vi "Untitled 2.vi"(0 "Data IN":T3={"App State"="", "Connect "=FALSE, "phandle out"=0, "Axis"=[], "S ramp"=30.0, "Acceleration"=100000.0, "Initial Speed"=10.0, "Normal Open / Close"=enum."Close", "Deceleration"=100000.0, "Creep"=30.0, "Speed"=1000.0, "X Axis"={"Operating State"="", "Current Position"=0.0, "Current Speed"=0.0, "Axis State"=0, "Angle"=0.0}, "Y Axis"={"Operating State"="", "Current Position"=0.0, "Current Speed"=0.0, "Axis State"=0, "Angle"=0.0}, "Distance"=0.0, "Direct of movement"=enum."Forward", "Move Method"=enum."Continue", "Move Mode"=enum."Relative", "Angle"=enum."0", "Times"=0, "Start Time"=0.0, "Step Flag"=FALSE, "x  dist"=[], "y dist"=[], "x angle array"=[], "y angle array"=[], "index"=0.0, "big motion angle"=0.0, "big angle"=[], "xy dy speed table"=[], "x dy speed table"=[], "y dy speed table"=[], "x dy time"=[], "y dy time"=[], "xy dy time"=[], "dy Path  "=[]}, 1 "Axis":enum16{"X", "Y", "X+Y"}(ring), 3 "Rotate":bool, 5 "dynamic":bool, 9 "Array 2":T2(array[cluster]), 11 "error IN":errorcluster, 12 "DYNAMIC":T1(array[cluster]), 13 "DYNAMIC 2":T1(array[cluster]), 14 "Speed":dbl=1.0 format="%#_13g") -> (4 "Data OUT":T3={"App State"="", "Connect "=FALSE, "phandle out"=0, "Axis"=[], "S ramp"=30.0, "Acceleration"=100000.0, "Initial Speed"=10.0, "Normal Open / Close"=enum."Close", "Deceleration"=100000.0, "Creep"=30.0, "Speed"=1000.0, "X Axis"={"Operating State"="", "Current Position"=0.0, "Current Speed"=0.0, "Axis State"=0, "Angle"=0.0}, "Y Axis"={"Operating State"="", "Current Position"=0.0, "Current Speed"=0.0, "Axis State"=0, "Angle"=0.0}, "Distance"=0.0, "Direct of movement"=enum."Forward", "Move Method"=enum."Continue", "Move Mode"=enum."Relative", "Angle"=enum."0", "Times"=0, "Start Time"=0.0, "Step Flag"=FALSE, "x  dist"=[], "y dist"=[], "x angle array"=[], "y angle array"=[], "index"=0.0, "big motion angle"=0.0, "big angle"=[], "xy dy speed table"=[], "x dy speed table"=[], "y dy speed table"=[], "x dy time"=[], "y dy time"=[], "xy dy time"=[], "dy Path  "=[]}, 15 "error out":errorcluster)   [LabVIEW 2015]
uses:
  Typedef/Data2.ctl
  zauxdll-2014/zauxdll.lvlib
panel:
  out "y angle array":i32[][](array[numeric])
  out "x angle array":i32[][](array[numeric])
  # "m"
  # "m"
  # "m"
  # "m"
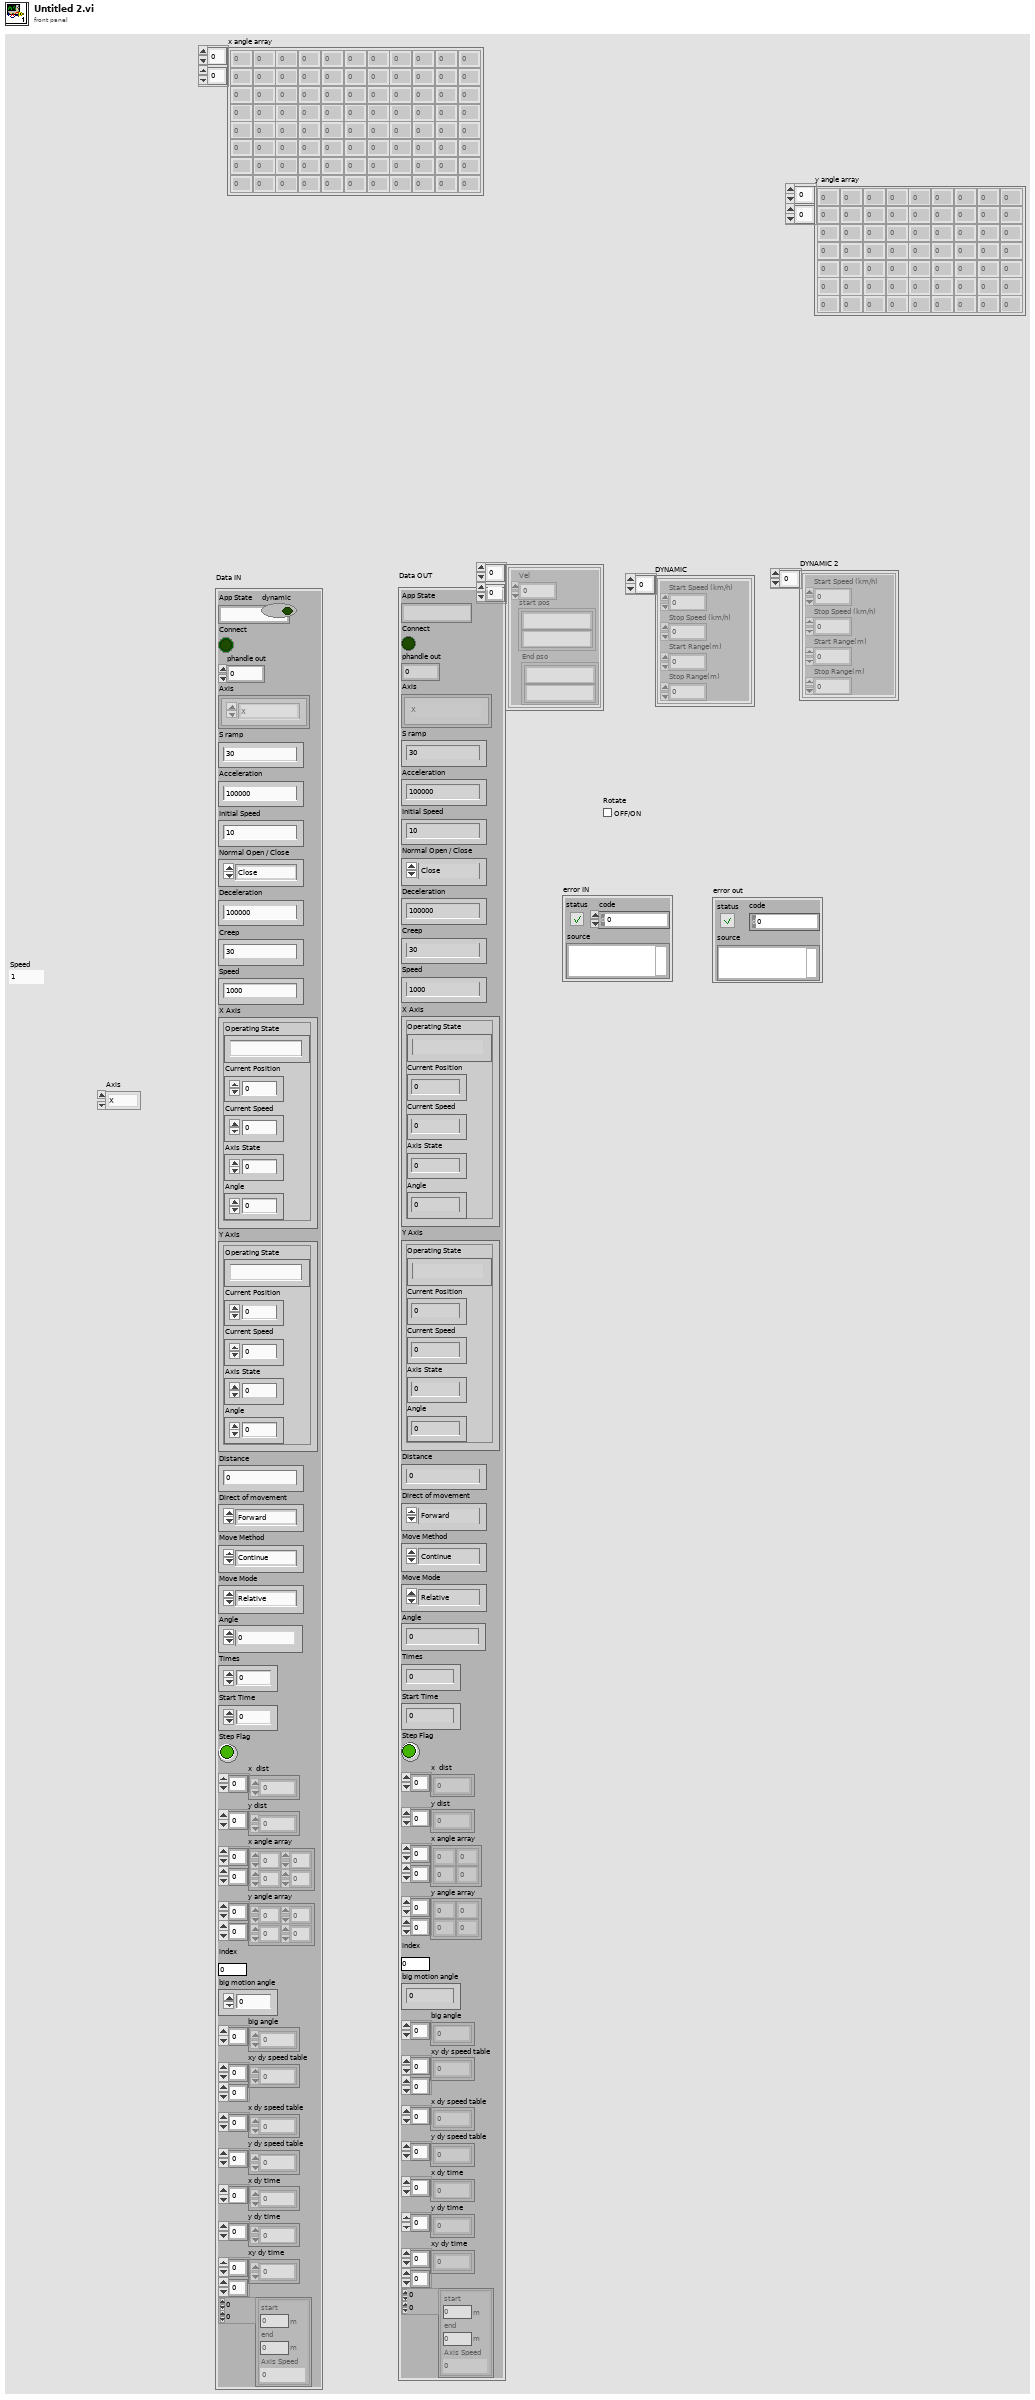
[diagram p1: front panel]
types:
  T1 = cluster{"Start Speed (km/h)":dbl, "Stop Speed (km/h) ":dbl, "Start Range(m)":dbl, "Stop Range(m)":dbl}[]
  T2 = cluster{"Vel":dbl, "start pos":cluster{string, string}, "End pso":cluster{string, string}}[][]
  T3 = typedef "Data2.ctl" = cluster{"App State":string, "Connect ":bool, "phandle out":u32, "Axis":enum16{"X", "Y", "X+Y"}[], "S ramp":dbl, "Acceleration":dbl, "Initial Speed":dbl, "Normal Open / Close":enum16{"Open", "Close"}, "Deceleration":dbl, "Creep":dbl, "Speed":dbl, "X Axis":cluster{"Operating State":string, "Current Position":dbl, "Current Speed":dbl, "Axis State":i32, "Angle":dbl}, "Y Axis":cluster{"Operating State":string, "Current Position":dbl, "Current Speed":dbl, "Axis State":i32, "Angle":dbl}, "Distance":dbl, "Direct of movement":enum16{"Forward", "Backward"}, "Move Method":enum16{"Continue", "Inching"}, "Move Mode":enum16{"Relative", "Absolute"}, "Angle":enum32{"0", "1", "10", "30", "34", "60", "90", "180", "-1", "-10"}, "Times":i32, "Start Time":dbl, "Step Flag":bool, "x  dist":dbl[], "y dist":dbl[], "x angle array":i32[][], "y angle array":i32[][], "index":dbl, "big motion angle":dbl, "big angle":dbl[], "xy dy speed table":dbl[][], "x dy speed table":dbl[], "y dy speed table":dbl[], "x dy time":dbl[], "y dy time":dbl[], "xy dy time":dbl[][], "dy Path  ":cluster{"end":dbl, "start":dbl, "Axis Speed":dbl}[][]}
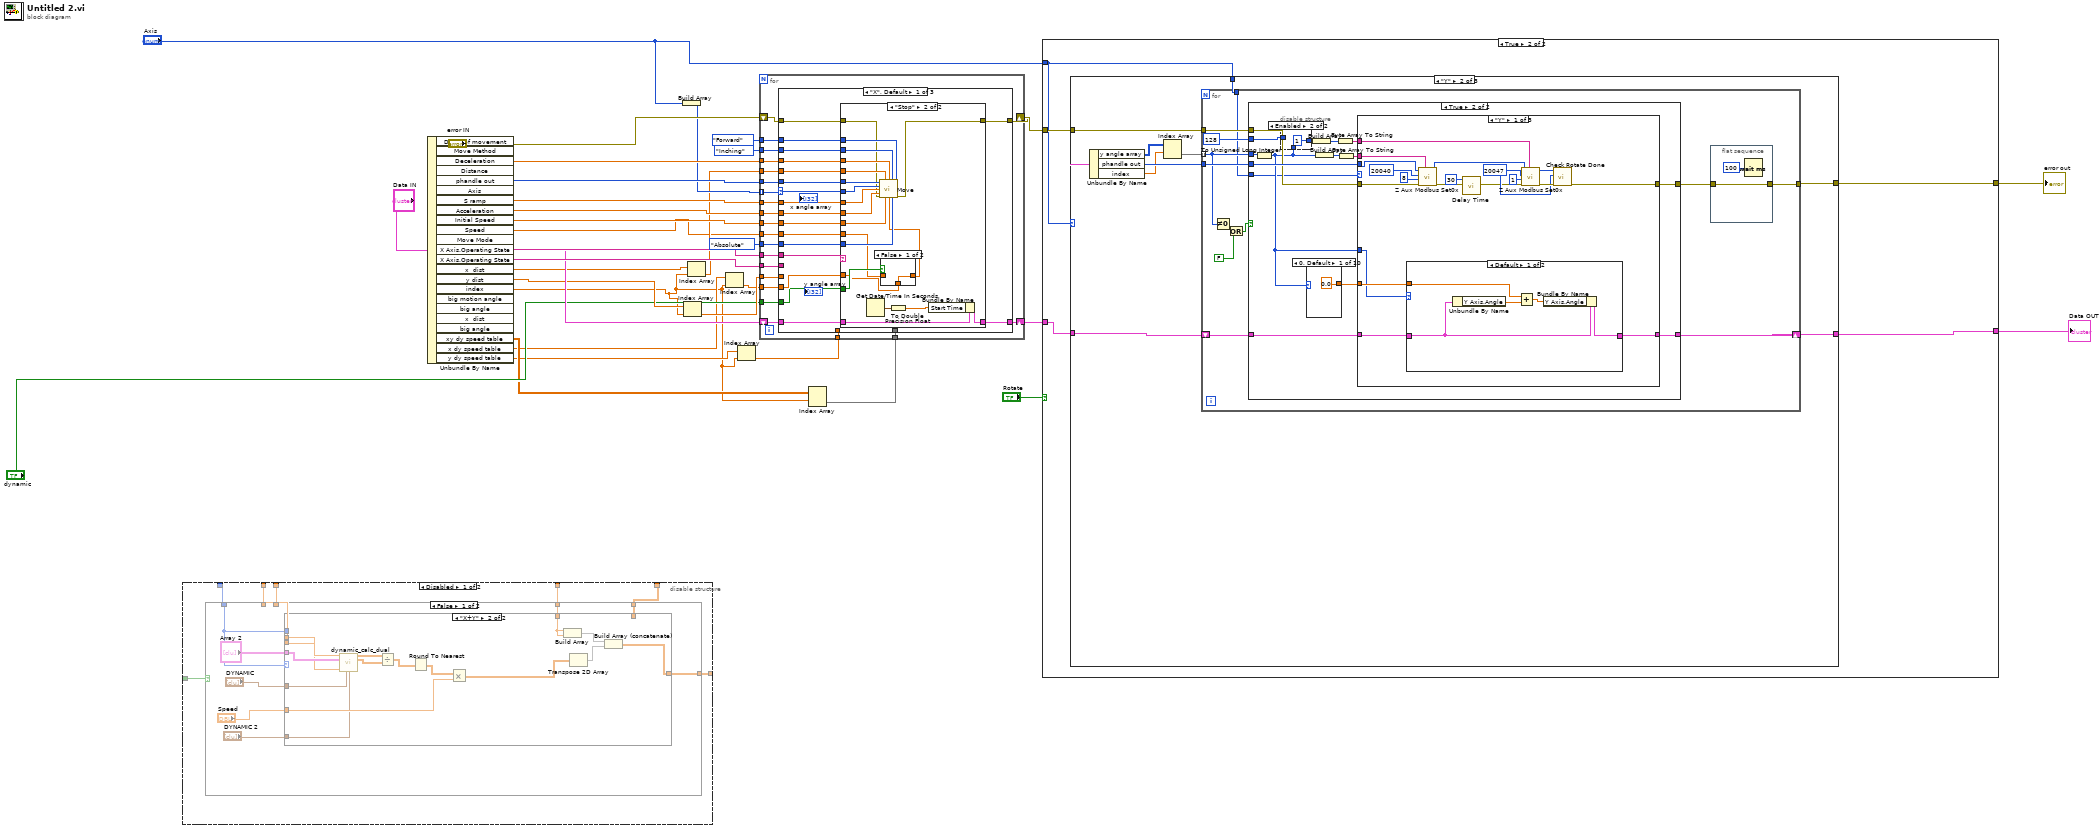
[diagram p0: block diagram]
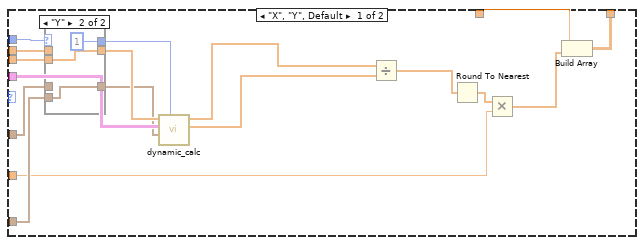
[diagram p2: hidden frame]
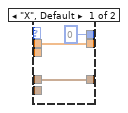
[diagram p3: hidden frame]
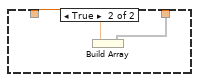
[diagram p4: hidden frame]
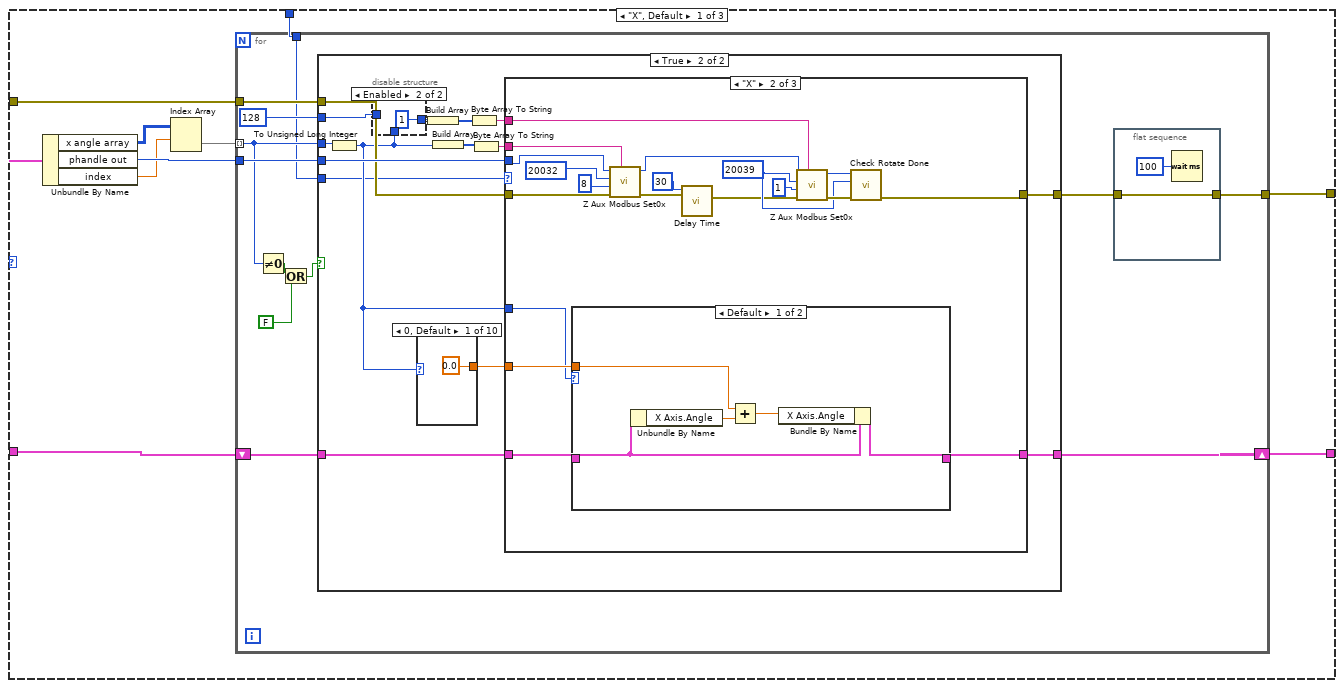
[diagram p7: hidden frame]
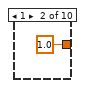
[diagram p9: hidden frame]
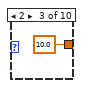
[diagram p10: hidden frame]
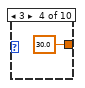
[diagram p11: hidden frame]
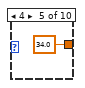
[diagram p12: hidden frame]
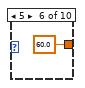
[diagram p13: hidden frame]
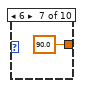
[diagram p14: hidden frame]
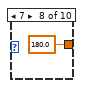
[diagram p15: hidden frame]
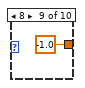
[diagram p16: hidden frame]
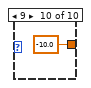
[diagram p17: hidden frame]
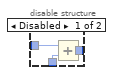
[diagram p18: hidden frame]
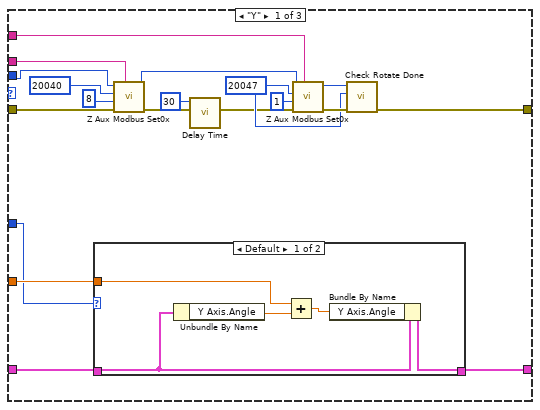
[diagram p19: hidden frame]
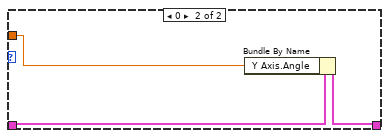
[diagram p20: hidden frame]
diagram:
  n1 = disable-structure shown="Disabled" {
    disable-tunnel: _ -> [w39 _]
    disable-tunnel: _ -> [w38 _]
    disable-tunnel: _ -> [w37 _]
    disable-tunnel: _ -> [w36 _]
    disable-tunnel: _ -> [w35 _]
    disable-tunnel: [w34 _] -> _
    disable-tunnel: [w33 _] -> _
    frame Disabled {
      n2 = case shown="False" w39 {
        tunnel: w38 -> [w43 _]
        tunnel: w37 -> [w49 w89]
        tunnel: [w48 w88] -> w34
        tunnel: w36 -> [w45 _]
        tunnel: w35 -> [w44 _]
        tunnel: [w41 _] -> w33
        frame False {
          n3 = case shown="\"X+Y\"" w43 {
            tunnel: w49 -> [w62 w78]
            tunnel: [w61 _] -> w48
            tunnel: "DYNAMIC" -> [w54 w74]
            tunnel: "Array 2" -> [w60 w87]
            tunnel: w45 -> [w58 w86]
            tunnel: w44 -> [w57 w85]
            tunnel: w43 -> [w59 _]
            tunnel: "Speed" -> [w51 w80]
            tunnel: [_ w79] -> w41
            tunnel: "DYNAMIC 2" -> [w53 w73]
            frame "X", "Y", Default {
              n4 = case shown="\"Y\"" w59 {
                tunnel: w58 -> [w69 _]
                tunnel: w57 -> [_ w72]
                tunnel: [w69 w72] -> w56
                tunnel: [0 1] -> w55
                tunnel: w54 -> [w67 _]
                tunnel: w53 -> [_ w70]
                tunnel: [w67 w70] -> w52
                frame "X", Default {
                }
                frame "Y" {
                }
              }
              n5 = call "dynamic_calc.vi"("index (row)"=w55, "DYNAMIC"=w52, "Array 2"=w60, "x  dist"=w56) -> ("time"=w64:dbl[], "Array"=w63:dbl[])  [unwired: 5 in, 1 out]
              n6 = Divide(x=w63, y=w64) -> (x/y=w50:dbl[])
              n7 = Round To Nearest(number=w50) -> (nearest integer value=w65:dbl[])
              n8 = Multiply(x=w65, y=w51) -> (x*y=w66:dbl[])
              n9 = Build Array(w62, w66) -> (w61:dbl[][])
            }
            frame "X+Y" {
              n10 = call "dynamic_calc_dual.vi"("x  dist"=w86, "Array 2"=w87, "y  dist"=w85, "DYNAMIC"=w74, "DYNAMIC 2"=w73) -> ("dist"=w84:dbl[][], "time"=w83:dbl[][])  [unwired: 9 in]
              n11 = Divide(x=w84, y=w83) -> (x/y=w82:dbl[][])
              n12 = Round To Nearest(number=w82) -> (nearest integer value=w81:dbl[][])
              n13 = Multiply(x=w81, y=w80) -> (x*y=w77:dbl[][])
              n14 = Build Array(w78, w78) -> (w75:void[])
              n15 = Transpose 2D Array(2D array=w77) -> (transposed array=w76:dbl[][])
              n16 = Build Array (concatenate)(w75, w76) -> (w79:dbl[][])
            }
          }
        }
        frame True {
          n17 = Build Array(w89) -> (w88:void[])
        }
      }
    }
    frame Enabled {
    }
  }
  n18 = Unbundle By Name("Data IN") -> ("Deceleration"=w28:dbl, "phandle out"=w32:u32, "S ramp"=w31:dbl, "Acceleration"=w30:dbl, "Initial Speed"=w29:dbl, "Speed"=w10:dbl, "X Axis.Operating State"=w27:string, "X Axis.Operating State"=w26:string, "x  dist"=w7:dbl[], "y dist"=w9:dbl[], "index"=w2:dbl, "xy dy speed table"=w5:dbl[][], "x dy speed table"=w4:dbl[], "y dy speed table"=w3:dbl[])  [unwired: 9 out]
  n19 = Build Array("Axis") -> (w16:enum16{"X", "Y", "X+Y"}[])
  n20 = Index Array(array=w9, index=w2) -> (element=w15:dbl)
  n21 = Index Array(array=w7, index=w2) -> (element=w13:dbl)
  n22 = Index Array(array=w4, index=w2) -> (element=w12:dbl)
  n23 = Index Array(array=w3, index=w2) -> (element=w1:dbl)
  n24 = Index Array(array=w5, index (row)=w2) -> (element=w8:dbl[])  [unwired: 1 in]
  n25 = for {
    tunnel: w32 -> [w111]
    tunnel: w31 -> [w110]
    tunnel: w30 -> [w109]
    tunnel: w29 -> [w108]
    tunnel: w10 -> [w107]
    tunnel: enum16{"Continue", "Inching"}."Inching" ("Move Method") -> [w106]
    tunnel: w28 -> [w105]
    tunnel: w16 -> [w104] mode=indexing
    tunnel: w13 -> [w103]
    tunnel: enum16{"Forward", "Backward"}."Forward" ("Direct of movement") -> [w102]
    tunnel: enum16{"Relative", "Absolute"}."Absolute" ("Move Mode") -> [w101]
    tunnel: w27 -> [w100]
    tunnel: w26 -> [w99]
    shift-right: [w97] -> w23
    shift-left: "Data IN" -> [w98]
    shift-right: [w95] -> w22
    shift-left: "error IN" -> [w96]
    tunnel: w15 -> [w94]
    tunnel: w12 -> [w93]
    tunnel: "dynamic" -> [w92]
    tunnel: w8 -> [w91]
    tunnel: w1 -> [w90]
    n26 = case shown="\"X\", Default" w104 {
      selector: w104 -> [w122 w165 _]
      tunnel: w111 -> [w129 w171 w219]
      tunnel: w110 -> [w128 w170 w218]
      tunnel: w109 -> [w127 w169 w217]
      tunnel: w108 -> [w126 w168 w216]
      tunnel: w107 -> [w125 w167 w215]
      tunnel: w106 -> [w124 w166 w214]
      tunnel: w105 -> [w123 w156 w213]
      tunnel: w103 -> [w120 _ w200]
      tunnel: w102 -> [w121 w164 w212]
      tunnel: w101 -> [w119 w163 w211]
      tunnel: w100 -> [w118 _ w210]
      tunnel: w99 -> [_ w162 w208]
      tunnel: w98 -> [w117 w161 w204]
      tunnel: [w116 w160 w203] -> w97
      tunnel: w96 -> [w115 w159 w202]
      tunnel: [w114 w158 w201] -> w95
      tunnel: w94 -> [_ w157 w199]
      tunnel: w93 -> [w113 _ _]
      tunnel: w92 -> [w112 w155 w197]
      tunnel: w91 -> [_ _ w196]
      tunnel: w90 -> [_ w154 _]
      frame "X", Default {
        n27 = case shown="\"Stop\"" w118 {
          tunnel: w129 -> [_ w151]
          tunnel: w128 -> [_ w150]
          tunnel: w127 -> [_ w149]
          tunnel: w126 -> [_ w148]
          tunnel: w125 -> [_ w134]
          tunnel: w124 -> [_ w147]
          tunnel: w123 -> [_ w146]
          tunnel: w122 -> [_ w145]
          tunnel: w121 -> [_ w144]
          tunnel: w120 -> [_ w143]
          tunnel: w119 -> [_ w142]
          tunnel: w117 -> [w131 w141]
          tunnel: [w131 w140] -> w116
          tunnel: w115 -> [w130 w137]
          tunnel: [w130 w136] -> w114
          tunnel: w113 -> [_ w132]
          tunnel: w112 -> [_ w135]
          frame "False", Default {
          }
          frame "Stop" {
            n28 = Get Date/Time In Seconds() -> (seconds since 1Jan1904=w139:timestamp)
            n29 = case shown="False" w135 {
              tunnel: w134 -> [_ w153]
              tunnel: [w152 w153] -> w133
              tunnel: w132 -> [w152 _]
              frame False {
              }
              frame True {
              }
            }
            n30 = call "Move.vi"("handle"=w151, "Distance"=w143, "Decel"=w146, "Move Method"=w147, "Direct of movement"=w144, "Axis"=w145, "Sramp"=w150, "Accel"=w149, "error in (no error)"=w137, "Lspeed"=w148, "Speed"=w133, "Move Mode"=w142) -> ("error out"=w136:errorcluster)  [unwired: 3 in]
            n31 = To Double Precision Float(number=w139) -> (double precision float=w138:dbl)
            n32 = Bundle By Name(cluster=w141, "Start Time"=w138) -> (w140:T3)
          }
        }
      }
      frame "Y" {
        n33 = case shown="\"Stop\"" w162 {
          tunnel: w171 -> [_ w193]
          tunnel: w170 -> [_ w192]
          tunnel: w169 -> [_ w191]
          tunnel: w168 -> [_ w190]
          tunnel: w167 -> [_ w176]
          tunnel: w166 -> [_ w189]
          tunnel: w156 -> [_ w188]
          tunnel: w165 -> [_ w187]
          tunnel: w164 -> [_ w186]
          tunnel: w157 -> [_ w185]
          tunnel: w163 -> [_ w184]
          tunnel: w161 -> [w173 w181]
          tunnel: [w173 w180] -> w160
          tunnel: w159 -> [w172 w179]
          tunnel: [w172 w178] -> w158
          tunnel: w154 -> [_ w174]
          tunnel: w155 -> [_ w177]
          frame "False", Default {
          }
          frame "Stop" {
            n34 = Get Date/Time In Seconds() -> (seconds since 1Jan1904=w183:timestamp)
            n35 = case shown="False" w177 {
              tunnel: w176 -> [_ w195]
              tunnel: [w194 w195] -> w175
              tunnel: w174 -> [w194 _]
              frame False {
              }
              frame True {
              }
            }
            n36 = To Double Precision Float(number=w183) -> (double precision float=w182:dbl)
            n37 = call "Move.vi"("handle"=w193, "Distance"=w185, "Decel"=w188, "Move Method"=w189, "Direct of movement"=w186, "Axis"=w187, "Sramp"=w192, "Accel"=w191, "error in (no error)"=w179, "Lspeed"=w190, "Speed"=w175, "Move Mode"=w184) -> ("error out"=w178:errorcluster)  [unwired: 3 in]
            n38 = Bundle By Name(cluster=w181, "Start Time"=w182) -> (w180:T3)
          }
        }
      }
      frame "X+Y" {
        w209 = "Stop" ("y")
        n39 = Build Array(w200, w199) -> (w198:dbl[])
        n40 = Equal?(x=w210, y=w209) -> (x = y?=w207:bool)
        n41 = Equal?(x=w209, y=w208) -> (x = y?=w205:bool)
        n42 = And(x=w207, y=w205) -> (x .and. y?=w206:bool)
        n43 = case shown="True" w206 {
          tunnel: w219 -> [_ w241]
          tunnel: w218 -> [_ w240]
          tunnel: w217 -> [_ w239]
          tunnel: w216 -> [_ w238]
          tunnel: w215 -> [_ w224]
          tunnel: w214 -> [_ w237]
          tunnel: w213 -> [_ w236]
          tunnel: w198 -> [_ w234]
          tunnel: w212 -> [_ w233]
          tunnel: w211 -> [_ w232]
          tunnel: w204 -> [w221 w231]
          tunnel: [w221 w230] -> w203
          tunnel: w202 -> [w220 w227]
          tunnel: [w220 w226] -> w201
          tunnel: w197 -> [_ w225]
          tunnel: w196 -> [_ w222]
          frame False {
          }
          frame True {
            n44 = case shown="False" w225 {
              tunnel: w224 -> [_ w244]
              tunnel: [w242 w243] -> w223
              tunnel: w222 -> [w242 _]
              frame False {
              }
              frame True {
                n45 = Build Array(w244, w244) -> (w243:dbl[])
              }
            }
            n46 = Get Date/Time In Seconds() -> (seconds since 1Jan1904=w229:timestamp)
            n47 = To Double Precision Float(number=w229) -> (double precision float=w228:dbl)
            n48 = for {
              tunnel: w241 -> [w257]
              tunnel: w240 -> [w256]
              tunnel: w239 -> [w255]
              tunnel: w238 -> [w254]
              tunnel: w223 -> [w253] mode=indexing
              tunnel: w237 -> [w252]
              tunnel: w236 -> [w251]
              tunnel: i32[] [0, 1] -> [w250] mode=indexing
              tunnel: w234 -> [w249] mode=indexing
              tunnel: w233 -> [w248]
              tunnel: w232 -> [w247]
              tunnel: w227 -> [w246]
              tunnel: [w245] -> w226
              n49 = call "Move.vi"("handle"=w257, "Distance"=w249, "Decel"=w251, "Move Method"=w252, "Direct of movement"=w248, "Axis"=w250, "Sramp"=w256, "Accel"=w255, "error in (no error)"=w246, "Lspeed"=w254, "Speed"=w253, "Move Mode"=w247) -> ("error out"=w245:errorcluster)  [unwired: 3 in]
            }
            n50 = Bundle By Name(cluster=w231, "Start Time"=w228) -> (w230:T3)
          }
        }
      }
    }
  }
  n51 = case shown="True" "Rotate" {
    tunnel: w23 -> [w258 w264]
    tunnel: w22 -> [w259 w263]
    tunnel: [w259 w262] -> w21
    tunnel: [w258 w261] -> w20
    tunnel: "Axis" -> [_ w260]
    frame False {
    }
    frame True {
      n52 = case shown="\"Y\"" w260 {
        tunnel: w264 -> [w271 w411 w552]
        tunnel: w263 -> [w270 w410 w556]
        tunnel: [w269 w409 w548] -> w262
        tunnel: [w268 w408 w550] -> w261
        tunnel: w260 -> [w267 w407 w555]
        frame "X", Default {
          n53 = Unbundle By Name(w271) -> ("x angle array"=w266:i32[][], "phandle out"=w273:u32, "index"=w265:dbl)
          n54 = Index Array(array=w266, index (row)=w265) -> (element=w272:i32[])  [unwired: 1 in]
          n55 = for {
            tunnel: w273 -> [w281]
            tunnel: w270 -> [w285]
            tunnel: w272 -> [w280] mode=indexing
            shift-right: [w282] -> w268
            shift-left: w271 -> [w283]
            tunnel: [w276] -> w269
            tunnel: w267 -> [w274]
            n56 = Not Equal To 0?(x=w280) -> (x != 0?=w278:bool)
            n57 = Or(x=w278, y=FALSE) -> (x .or. y?=w279:bool)
            n58 = case shown="True" w279 {
              tunnel: w281 -> [_ w304]
              tunnel: w285 -> [w289 w303]
              tunnel: u32 128 -> [_ w302]
              tunnel: w283 -> [w288 w296]
              tunnel: w280 -> [_ w295]
              tunnel: [w288 w294] -> w282
              tunnel: [w289 w293] -> w277
              tunnel: w274 -> [_ w290]
              frame False {
              }
              frame True {
                n59 = To Unsigned Long Integer(number=w295) -> (unsigned 32bit integer=w291:u32)
                n60 = disable-structure shown="Enabled" {
                  disable-tunnel: w302 -> [w317 _]
                  disable-tunnel: [w316 u32 1] -> w301
                  disable-tunnel: w291 -> [w315 _]
                  frame Disabled {
                    n61 = Add(x=w317, y=w315) -> (x+y=w316:u32)
                  }
                  frame Enabled {
                  }
                }
                n62 = case shown="0, Default" w291 {
                  tunnel: [0.0 1.0 10.0 30.0 34.0 60.0 90.0 180.0 -1.0 -10.0] -> w297
                  frame 0, Default {
                  }
                  frame 1 {
                  }
                  frame 2 {
                  }
                  frame 3 {
                  }
                  frame 4 {
                  }
                  frame 5 {
                  }
                  frame 6 {
                  }
                  frame 7 {
                  }
                  frame 8 {
                  }
                  frame 9 {
                  }
                }
                n63 = Build Array(w301) -> (w300:u32[])
                n64 = Build Array(w291) -> (w292:u32[])
                n65 = Byte Array To String(unsigned byte array=w300) -> (string=w299:string)
                n66 = Byte Array To String(unsigned byte array=w292) -> (string=w298:string)
                n67 = case shown="\"X\"" w290 {
                  tunnel: w304 -> [w334 w361 w388]
                  tunnel: w299 -> [w335 w362 w389]
                  tunnel: w298 -> [w333 w360 w387]
                  tunnel: w303 -> [w328 w355 w384]
                  tunnel: [w323 w350 w380] -> w293
                  tunnel: w296 -> [w322 w349 w377]
                  tunnel: [w321 w348 w376] -> w294
                  tunnel: w297 -> [w320 w347 w373]
                  tunnel: w291 -> [w319 w346 _]
                  frame "Y" {
                    w329 = u16 20047 ("start")
                    n68 = case shown="Default" w319 {
                      tunnel: w322 -> [w342 w345]
                      tunnel: [w341 w344] -> w321
                      tunnel: w320 -> [w338 w343]
                      frame Default {
                        n69 = Unbundle By Name(w342) -> ("Y Axis.Angle"=w339:dbl)
                        n70 = Add(x=w338, y=w339) -> (x+y=w340:dbl)
                        n71 = Bundle By Name(cluster=w342, "Y Axis.Angle"=w340) -> (w341:T3)
                      }
                      frame 0 {
                        n72 = Bundle By Name(cluster=w345, "Y Axis.Angle"=w343) -> (w344:T3)
                      }
                    }
                    n73 = call "Z Aux Modbus Set0x.vi"("pdata"=w333, "error in (no error)"=w328, "inum"=u16 8, "start"=u16 20040, "handle"=w334) -> ("error out"=w326:errorcluster, "handle out"=w327:u32)  [unwired: 3 in, 2 out]
                    n74 = call "Delay Time.vi"("error in (no error)"=w326, "Delay(ms)"=u32 30) -> ("error out"=w324:errorcluster)  [unwired: 9 in]
                    n75 = call "Z Aux Modbus Set0x.vi"("pdata"=w335, "error in (no error)"=w324, "inum"=u16 1, "start"=w329, "handle"=w327) -> ("error out"=w337:errorcluster, "handle out"=w336:u32)  [unwired: 3 in, 2 out]
                    n76 = call "Check Rotate Done.vi"("error in (no error)"=w337, "start"=w329, "phandle in"=w336) -> ("error out"=w323:errorcluster)  [unwired: 8 in]
                  }
                  frame "X" {
                    w356 = u16 20039 ("start")
                    n77 = case shown="Default" w346 {
                      tunnel: w349 -> [w369 w372]
                      tunnel: [w368 w371] -> w348
                      tunnel: w347 -> [w365 w370]
                      frame Default {
                        n78 = Unbundle By Name(w369) -> ("X Axis.Angle"=w367:dbl)
                        n79 = Add(x=w365, y=w367) -> (x+y=w366:dbl)
                        n80 = Bundle By Name(cluster=w369, "X Axis.Angle"=w366) -> (w368:T3)
                      }
                      frame 0 {
                        n81 = Bundle By Name(cluster=w372, "X Axis.Angle"=w370) -> (w371:T3)
                      }
                    }
                    n82 = call "Z Aux Modbus Set0x.vi"("pdata"=w360, "error in (no error)"=w355, "inum"=u16 8, "start"=u16 20032, "handle"=w361) -> ("error out"=w353:errorcluster, "handle out"=w354:u32)  [unwired: 3 in, 2 out]
                    n83 = call "Delay Time.vi"("error in (no error)"=w353, "Delay(ms)"=u32 30) -> ("error out"=w351:errorcluster)  [unwired: 9 in]
                    n84 = call "Z Aux Modbus Set0x.vi"("pdata"=w362, "error in (no error)"=w351, "inum"=u16 1, "start"=w356, "handle"=w354) -> ("error out"=w364:errorcluster, "handle out"=w363:u32)  [unwired: 3 in, 2 out]
                    n85 = call "Check Rotate Done.vi"("error in (no error)"=w364, "start"=w356, "phandle in"=w363) -> ("error out"=w350:errorcluster)  [unwired: 8 in]
                  }
                  frame "X+Y" {
                    n86 = Unbundle By Name(w377) -> ("X Axis.Angle"=w379:dbl, "Y Axis.Angle"=w378:dbl)
                    n87 = for {
                      tunnel: w387 -> [w403]
                      shift-right: [w402] -> w382
                      shift-left: w388 -> [w404]
                      tunnel: i32[] [20032, 20040] -> [w400] mode=indexing
                      tunnel: w384 -> [w399]
                      tunnel: [w398] -> w383
                      n88 = call "Z Aux Modbus Set0x.vi"("pdata"=w403, "error in (no error)"=w399, "inum"=u16 8, "start"=w400, "handle"=w404) -> ("error out"=w398:errorcluster, "handle out"=w402:u32)  [unwired: 3 in, 2 out]
                    }
                    n89 = call "Delay Time.vi"("error in (no error)"=w383) -> ("error out"=w381:errorcluster)  [unwired: 10 in]
                    n90 = Add(x=w373, y=w379) -> (x+y=w375:dbl)
                    n91 = Add(x=w378, y=w373) -> (x+y=w374:dbl)
                    n92 = for {
                      tunnel: w389 -> [w395]
                      tunnel: w382 -> [w394]
                      tunnel: i32[] [20039, 20047] -> [w392] mode=indexing
                      tunnel: w381 -> [w391]
                      tunnel: [w390] -> w380
                      n93 = call "Z Aux Modbus Set0x.vi"("pdata"=w395, "error in (no error)"=w391, "inum"=u16 1, "start"=w392, "handle"=w394) -> ("error out"=w397:errorcluster, "handle out"=w396:u32)  [unwired: 3 in, 2 out]
                      n94 = call "Check Rotate Done.vi"("error in (no error)"=w397, "start"=w392, "phandle in"=w396) -> ("error out"=w390:errorcluster)  [unwired: 8 in]
                    }
                    n95 = Bundle By Name(cluster=w377, "X Axis.Angle"=w375, "Y Axis.Angle"=w374) -> (w376:T3)
                  }
                }
              }
            }
            n96 = flat-sequence {
              tunnel: w277 -> [w287]
              tunnel: [w287] -> w276
              frame #0 {
                n97 = Wait (ms)(milliseconds to wait=u32 100) -> ()  [unwired: 1 out]
              }
            }
          }
        }
        frame "Y" {
          n98 = Unbundle By Name(w411) -> ("y angle array"=w406:i32[][], "phandle out"=w413:u32, "index"=w405:dbl)
          n99 = Index Array(array=w406, index (row)=w405) -> (element=w412:i32[])  [unwired: 1 in]
          n100 = for {
            tunnel: w413 -> [w421]
            tunnel: w410 -> [w425]
            tunnel: w412 -> [w420] mode=indexing
            shift-right: [w422] -> w408
            shift-left: w411 -> [w423]
            tunnel: [w416] -> w409
            tunnel: w407 -> [w414]
            n101 = Not Equal To 0?(x=w420) -> (x != 0?=w418:bool)
            n102 = Or(x=w418, y=FALSE) -> (x .or. y?=w419:bool)
            n103 = case shown="True" w419 {
              tunnel: w421 -> [_ w444]
              tunnel: w425 -> [w429 w443]
              tunnel: u32 128 -> [_ w442]
              tunnel: w423 -> [w428 w436]
              tunnel: w420 -> [_ w435]
              tunnel: [w428 w434] -> w422
              tunnel: [w429 w433] -> w417
              tunnel: w414 -> [_ w430]
              frame False {
              }
              frame True {
                n104 = To Unsigned Long Integer(number=w435) -> (unsigned 32bit integer=w431:u32)
                n105 = disable-structure shown="Enabled" {
                  disable-tunnel: w442 -> [w457 _]
                  disable-tunnel: [w456 u32 1] -> w441
                  disable-tunnel: w431 -> [w455 _]
                  frame Disabled {
                    n106 = Add(x=w457, y=w455) -> (x+y=w456:u32)
                  }
                  frame Enabled {
                  }
                }
                n107 = case shown="0, Default" w431 {
                  tunnel: [0.0 1.0 10.0 30.0 34.0 60.0 90.0 180.0 -1.0 -10.0] -> w437
                  frame 0, Default {
                  }
                  frame 1 {
                  }
                  frame 2 {
                  }
                  frame 3 {
                  }
                  frame 4 {
                  }
                  frame 5 {
                  }
                  frame 6 {
                  }
                  frame 7 {
                  }
                  frame 8 {
                  }
                  frame 9 {
                  }
                }
                n108 = Build Array(w441) -> (w440:u32[])
                n109 = Build Array(w431) -> (w432:u32[])
                n110 = Byte Array To String(unsigned byte array=w440) -> (string=w439:string)
                n111 = Byte Array To String(unsigned byte array=w432) -> (string=w438:string)
                n112 = case shown="\"Y\"" w430 {
                  tunnel: w444 -> [w474 w501 w528]
                  tunnel: w439 -> [w475 w502 w529]
                  tunnel: w438 -> [w473 w500 w527]
                  tunnel: w443 -> [w468 w495 w524]
                  tunnel: [w463 w490 w520] -> w433
                  tunnel: w436 -> [w462 w489 w517]
                  tunnel: [w461 w488 w516] -> w434
                  tunnel: w437 -> [w460 w487 w513]
                  tunnel: w431 -> [w459 w486 _]
                  frame "Y" {
                    w469 = u16 20047 ("start")
                    n113 = case shown="Default" w459 {
                      tunnel: w462 -> [w482 w485]
                      tunnel: [w481 w484] -> w461
                      tunnel: w460 -> [w478 w483]
                      frame Default {
                        n114 = Unbundle By Name(w482) -> ("Y Axis.Angle"=w479:dbl)
                        n115 = Add(x=w478, y=w479) -> (x+y=w480:dbl)
                        n116 = Bundle By Name(cluster=w482, "Y Axis.Angle"=w480) -> (w481:T3)
                      }
                      frame 0 {
                        n117 = Bundle By Name(cluster=w485, "Y Axis.Angle"=w483) -> (w484:T3)
                      }
                    }
                    n118 = call "Z Aux Modbus Set0x.vi"("pdata"=w473, "error in (no error)"=w468, "inum"=u16 8, "start"=u16 20040, "handle"=w474) -> ("error out"=w466:errorcluster, "handle out"=w467:u32)  [unwired: 3 in, 2 out]
                    n119 = call "Delay Time.vi"("error in (no error)"=w466, "Delay(ms)"=u32 30) -> ("error out"=w464:errorcluster)  [unwired: 9 in]
                    n120 = call "Z Aux Modbus Set0x.vi"("pdata"=w475, "error in (no error)"=w464, "inum"=u16 1, "start"=w469, "handle"=w467) -> ("error out"=w477:errorcluster, "handle out"=w476:u32)  [unwired: 3 in, 2 out]
                    n121 = call "Check Rotate Done.vi"("error in (no error)"=w477, "start"=w469, "phandle in"=w476) -> ("error out"=w463:errorcluster)  [unwired: 8 in]
                  }
                  frame "X" {
                    w496 = u16 20039 ("start")
                    n122 = case shown="0" w486 {
                      tunnel: w489 -> [w509 w512]
                      tunnel: [w508 w511] -> w488
                      tunnel: w487 -> [w505 w510]
                      frame Default {
                        n123 = Unbundle By Name(w509) -> ("X Axis.Angle"=w507:dbl)
                        n124 = Add(x=w505, y=w507) -> (x+y=w506:dbl)
                        n125 = Bundle By Name(cluster=w509, "X Axis.Angle"=w506) -> (w508:T3)
                      }
                      frame 0 {
                        n126 = Bundle By Name(cluster=w512, "X Axis.Angle"=w510) -> (w511:T3)
                      }
                    }
                    n127 = call "Z Aux Modbus Set0x.vi"("pdata"=w500, "error in (no error)"=w495, "inum"=u16 8, "start"=u16 20032, "handle"=w501) -> ("error out"=w493:errorcluster, "handle out"=w494:u32)  [unwired: 3 in, 2 out]
                    n128 = call "Delay Time.vi"("error in (no error)"=w493, "Delay(ms)"=u32 30) -> ("error out"=w491:errorcluster)  [unwired: 9 in]
                    n129 = call "Z Aux Modbus Set0x.vi"("pdata"=w502, "error in (no error)"=w491, "inum"=u16 1, "start"=w496, "handle"=w494) -> ("error out"=w504:errorcluster, "handle out"=w503:u32)  [unwired: 3 in, 2 out]
                    n130 = call "Check Rotate Done.vi"("error in (no error)"=w504, "start"=w496, "phandle in"=w503) -> ("error out"=w490:errorcluster)  [unwired: 8 in]
                  }
                  frame "X+Y" {
                    n131 = Unbundle By Name(w517) -> ("X Axis.Angle"=w519:dbl, "Y Axis.Angle"=w518:dbl)
                    n132 = for {
                      tunnel: w527 -> [w543]
                      shift-right: [w542] -> w522
                      shift-left: w528 -> [w544]
                      tunnel: i32[] [20032, 20040] -> [w540] mode=indexing
                      tunnel: w524 -> [w539]
                      tunnel: [w538] -> w523
                      n133 = call "Z Aux Modbus Set0x.vi"("pdata"=w543, "error in (no error)"=w539, "inum"=u16 8, "start"=w540, "handle"=w544) -> ("error out"=w538:errorcluster, "handle out"=w542:u32)  [unwired: 3 in, 2 out]
                    }
                    n134 = call "Delay Time.vi"("error in (no error)"=w523) -> ("error out"=w521:errorcluster)  [unwired: 10 in]
                    n135 = Add(x=w513, y=w519) -> (x+y=w515:dbl)
                    n136 = Add(x=w518, y=w513) -> (x+y=w514:dbl)
                    n137 = for {
                      tunnel: w529 -> [w535]
                      tunnel: w522 -> [w534]
                      tunnel: i32[] [20039, 20047] -> [w532] mode=indexing
                      tunnel: w521 -> [w531]
                      tunnel: [w530] -> w520
                      n138 = call "Z Aux Modbus Set0x.vi"("pdata"=w535, "error in (no error)"=w531, "inum"=u16 1, "start"=w532, "handle"=w534) -> ("error out"=w537:errorcluster, "handle out"=w536:u32)  [unwired: 3 in, 2 out]
                      n139 = call "Check Rotate Done.vi"("error in (no error)"=w537, "start"=w532, "phandle in"=w536) -> ("error out"=w530:errorcluster)  [unwired: 8 in]
                    }
                    n140 = Bundle By Name(cluster=w517, "X Axis.Angle"=w515, "Y Axis.Angle"=w514) -> (w516:T3)
                  }
                }
              }
            }
            n141 = flat-sequence {
              tunnel: w417 -> [w427]
              tunnel: [w427] -> w416
              frame #0 {
                n142 = Wait (ms)(milliseconds to wait=u32 100) -> ()  [unwired: 1 out]
              }
            }
          }
        }
        frame "X+Y" {
          n143 = Unbundle By Name(w552) -> ("x angle array"=w554:i32[][], "phandle out"=w546:u32, "index"=w545:dbl, "y angle array"=w553:i32[][])
          n144 = Index Array(array=w553, index (row)=w545) -> (element=w547:i32[])  [unwired: 1 in]
          n145 = Index Array(array=w554, index (row)=w545) -> (element=w557:i32[])  [unwired: 1 in]
          n146 = for {
            tunnel: w546 -> [w696]
            tunnel: w556 -> [w699]
            tunnel: w557 -> [w695] mode=indexing
            shift-right: [w689] -> w551
            shift-left: w552 -> [w697]
            tunnel: [w688] -> w549
            tunnel: w555 -> [w690]
            n147 = Not Equal To 0?(x=w695) -> (x != 0?=w693:bool)
            n148 = Or(x=w693, y=FALSE) -> (x .or. y?=w694:bool)
            n149 = case shown="True" w694 {
              tunnel: w696 -> [_ w718]
              tunnel: w699 -> [w703 w717]
              tunnel: u32 128 -> [_ w716]
              tunnel: w697 -> [w702 w710]
              tunnel: w695 -> [_ w709]
              tunnel: [w702 w708] -> w689
              tunnel: [w703 w707] -> w692
              tunnel: w690 -> [_ _]
              frame False {
              }
              frame True {
                n150 = To Unsigned Long Integer(number=w709) -> (unsigned 32bit integer=w705:u32)
                n151 = disable-structure shown="Enabled" {
                  disable-tunnel: w716 -> [w731 _]
                  disable-tunnel: [w730 u32 1] -> w715
                  disable-tunnel: w705 -> [w729 _]
                  frame Disabled {
                    n152 = Add(x=w731, y=w729) -> (x+y=w730:u32)
                  }
                  frame Enabled {
                  }
                }
                n153 = case shown="0, Default" w705 {
                  tunnel: [0.0 1.0 10.0 30.0 34.0 60.0 90.0 180.0 -1.0 -10.0] -> w711
                  frame 0, Default {
                  }
                  frame 1 {
                  }
                  frame 2 {
                  }
                  frame 3 {
                  }
                  frame 4 {
                  }
                  frame 5 {
                  }
                  frame 6 {
                  }
                  frame 7 {
                  }
                  frame 8 {
                  }
                  frame 9 {
                  }
                }
                n154 = Build Array(w715) -> (w714:u32[])
                n155 = Build Array(w705) -> (w706:u32[])
                n156 = Byte Array To String(unsigned byte array=w714) -> (string=w713:string)
                n157 = Byte Array To String(unsigned byte array=w706) -> (string=w712:string)
                n158 = case shown="\"X\"" enum16{"X", "Y", "X+Y"}."X" ("Axis") {
                  tunnel: w718 -> [w748 w775 w802]
                  tunnel: w713 -> [w749 w776 w803]
                  tunnel: w712 -> [w747 w774 w801]
                  tunnel: w717 -> [w742 w769 w798]
                  tunnel: [w737 w764 w794] -> w707
                  tunnel: w710 -> [w736 w763 w791]
                  tunnel: [w735 w762 w790] -> w708
                  tunnel: w711 -> [w734 w761 w787]
                  tunnel: w705 -> [w733 w760 _]
                  frame "Y" {
                    w743 = u16 20047 ("start")
                    n159 = case shown="0" w733 {
                      tunnel: w736 -> [w756 w759]
                      tunnel: [w755 w758] -> w735
                      tunnel: w734 -> [w752 w757]
                      frame Default {
                        n160 = Unbundle By Name(w756) -> ("X Axis.Angle"=w753:dbl)
                        n161 = Add(x=w752, y=w753) -> (x+y=w754:dbl)
                        n162 = Bundle By Name(cluster=w756, "X Axis.Angle"=w754) -> (w755:T3)
                      }
                      frame 0 {
                        n163 = Bundle By Name(cluster=w759, "X Axis.Angle"=w757) -> (w758:T3)
                      }
                    }
                    n164 = call "Z Aux Modbus Set0x.vi"("pdata"=w747, "error in (no error)"=w742, "inum"=u16 8, "start"=u16 20040, "handle"=w748) -> ("error out"=w740:errorcluster, "handle out"=w741:u32)  [unwired: 3 in, 2 out]
                    n165 = call "Delay Time.vi"("error in (no error)"=w740, "Delay(ms)"=u32 30) -> ("error out"=w738:errorcluster)  [unwired: 9 in]
                    n166 = call "Z Aux Modbus Set0x.vi"("pdata"=w749, "error in (no error)"=w738, "inum"=u16 1, "start"=w743, "handle"=w741) -> ("error out"=w751:errorcluster, "handle out"=w750:u32)  [unwired: 3 in, 2 out]
                    n167 = call "Check Rotate Done.vi"("error in (no error)"=w751, "start"=w743, "phandle in"=w750) -> ("error out"=w737:errorcluster)  [unwired: 8 in]
                  }
                  frame "X" {
                    w770 = u16 20039 ("start")
                    n168 = case shown="0" w760 {
                      tunnel: w763 -> [w783 w786]
                      tunnel: [w782 w785] -> w762
                      tunnel: w761 -> [w779 w784]
                      frame Default {
                        n169 = Unbundle By Name(w783) -> ("X Axis.Angle"=w781:dbl)
                        n170 = Add(x=w779, y=w781) -> (x+y=w780:dbl)
                        n171 = Bundle By Name(cluster=w783, "X Axis.Angle"=w780) -> (w782:T3)
                      }
                      frame 0 {
                        n172 = Bundle By Name(cluster=w786, "X Axis.Angle"=w784) -> (w785:T3)
                      }
                    }
                    n173 = call "Z Aux Modbus Set0x.vi"("pdata"=w774, "error in (no error)"=w769, "inum"=u16 8, "start"=u16 20032, "handle"=w775) -> ("error out"=w767:errorcluster, "handle out"=w768:u32)  [unwired: 3 in, 2 out]
                    n174 = call "Delay Time.vi"("error in (no error)"=w767, "Delay(ms)"=u32 30) -> ("error out"=w765:errorcluster)  [unwired: 9 in]
                    n175 = call "Z Aux Modbus Set0x.vi"("pdata"=w776, "error in (no error)"=w765, "inum"=u16 1, "start"=w770, "handle"=w768) -> ("error out"=w778:errorcluster, "handle out"=w777:u32)  [unwired: 3 in, 2 out]
                    n176 = call "Check Rotate Done.vi"("error in (no error)"=w778, "start"=w770, "phandle in"=w777) -> ("error out"=w764:errorcluster)  [unwired: 8 in]
                  }
                  frame "X+Y" {
                    n177 = Unbundle By Name(w791) -> ("X Axis.Angle"=w793:dbl, "Y Axis.Angle"=w792:dbl)
                    n178 = for {
                      tunnel: w801 -> [w817]
                      shift-right: [w816] -> w796
                      shift-left: w802 -> [w818]
                      tunnel: i32[] [20032, 20040] -> [w814] mode=indexing
                      tunnel: w798 -> [w813]
                      tunnel: [w812] -> w797
                      n179 = call "Z Aux Modbus Set0x.vi"("pdata"=w817, "error in (no error)"=w813, "inum"=u16 8, "start"=w814, "handle"=w818) -> ("error out"=w812:errorcluster, "handle out"=w816:u32)  [unwired: 3 in, 2 out]
                    }
                    n180 = call "Delay Time.vi"("error in (no error)"=w797) -> ("error out"=w795:errorcluster)  [unwired: 10 in]
                    n181 = Add(x=w787, y=w793) -> (x+y=w789:dbl)
                    n182 = Add(x=w792, y=w787) -> (x+y=w788:dbl)
                    n183 = for {
                      tunnel: w803 -> [w809]
                      tunnel: w796 -> [w808]
                      tunnel: i32[] [20039, 20047] -> [w806] mode=indexing
                      tunnel: w795 -> [w805]
                      tunnel: [w804] -> w794
                      n184 = call "Z Aux Modbus Set0x.vi"("pdata"=w809, "error in (no error)"=w805, "inum"=u16 1, "start"=w806, "handle"=w808) -> ("error out"=w811:errorcluster, "handle out"=w810:u32)  [unwired: 3 in, 2 out]
                      n185 = call "Check Rotate Done.vi"("error in (no error)"=w811, "start"=w806, "phandle in"=w810) -> ("error out"=w804:errorcluster)  [unwired: 8 in]
                    }
                    n186 = Bundle By Name(cluster=w791, "X Axis.Angle"=w789, "Y Axis.Angle"=w788) -> (w790:T3)
                  }
                }
              }
            }
            n187 = flat-sequence {
              tunnel: w692 -> [w701]
              tunnel: [w701] -> w688
              frame #0 {
                n188 = Wait (ms)(milliseconds to wait=u32 100) -> ()  [unwired: 1 out]
              }
            }
          }
          n189 = for {
            tunnel: w546 -> [w564]
            tunnel: w549 -> [w568]
            tunnel: w547 -> [w563] mode=indexing
            shift-right: [w565] -> w550
            shift-left: w551 -> [w566]
            tunnel: [w559] -> w548
            n190 = Not Equal To 0?(x=w563) -> (x != 0?=w561:bool)
            n191 = Or(x=w561, y=FALSE) -> (x .or. y?=w562:bool)
            n192 = case shown="True" w562 {
              tunnel: w564 -> [_ w587]
              tunnel: w568 -> [w572 w586]
              tunnel: u32 128 -> [_ w585]
              tunnel: w566 -> [w571 w579]
              tunnel: w563 -> [_ w578]
              tunnel: [w571 w577] -> w565
              tunnel: [w572 w576] -> w560
              frame False {
              }
              frame True {
                n193 = To Unsigned Long Integer(number=w578) -> (unsigned 32bit integer=w574:u32)
                n194 = disable-structure shown="Enabled" {
                  disable-tunnel: w585 -> [w600 _]
                  disable-tunnel: [w599 u32 1] -> w584
                  disable-tunnel: w574 -> [w598 _]
                  frame Disabled {
                    n195 = Add(x=w600, y=w598) -> (x+y=w599:u32)
                  }
                  frame Enabled {
                  }
                }
                n196 = case shown="0, Default" w574 {
                  tunnel: [0.0 1.0 10.0 30.0 34.0 60.0 90.0 180.0 -1.0 -10.0] -> w580
                  frame 0, Default {
                  }
                  frame 1 {
                  }
                  frame 2 {
                  }
                  frame 3 {
                  }
                  frame 4 {
                  }
                  frame 5 {
                  }
                  frame 6 {
                  }
                  frame 7 {
                  }
                  frame 8 {
                  }
                  frame 9 {
                  }
                }
                n197 = Build Array(w584) -> (w583:u32[])
                n198 = Build Array(w574) -> (w575:u32[])
                n199 = Byte Array To String(unsigned byte array=w583) -> (string=w582:string)
                n200 = Byte Array To String(unsigned byte array=w575) -> (string=w581:string)
                n201 = case shown="\"Y\"" enum16{"X", "Y", "X+Y"}."Y" ("Axis") {
                  tunnel: w587 -> [w617 w644 w671]
                  tunnel: w582 -> [w618 w645 w672]
                  tunnel: w581 -> [w616 w643 w670]
                  tunnel: w586 -> [w611 w638 w667]
                  tunnel: [w606 w633 w663] -> w576
                  tunnel: w579 -> [w605 w632 w660]
                  tunnel: [w604 w631 w659] -> w577
                  tunnel: w580 -> [w603 w630 w656]
                  tunnel: w574 -> [w602 w629 _]
                  frame "Y" {
                    w612 = u16 20047 ("start")
                    n202 = case shown="Default" w602 {
                      tunnel: w605 -> [w625 w628]
                      tunnel: [w624 w627] -> w604
                      tunnel: w603 -> [w621 w626]
                      frame Default {
                        n203 = Unbundle By Name(w625) -> ("Y Axis.Angle"=w622:dbl)
                        n204 = Add(x=w621, y=w622) -> (x+y=w623:dbl)
                        n205 = Bundle By Name(cluster=w625, "Y Axis.Angle"=w623) -> (w624:T3)
                      }
                      frame 0 {
                        n206 = Bundle By Name(cluster=w628, "Y Axis.Angle"=w626) -> (w627:T3)
                      }
                    }
                    n207 = call "Z Aux Modbus Set0x.vi"("pdata"=w616, "error in (no error)"=w611, "inum"=u16 8, "start"=u16 20040, "handle"=w617) -> ("error out"=w609:errorcluster, "handle out"=w610:u32)  [unwired: 3 in, 2 out]
                    n208 = call "Delay Time.vi"("error in (no error)"=w609, "Delay(ms)"=u32 30) -> ("error out"=w607:errorcluster)  [unwired: 9 in]
                    n209 = call "Z Aux Modbus Set0x.vi"("pdata"=w618, "error in (no error)"=w607, "inum"=u16 1, "start"=w612, "handle"=w610) -> ("error out"=w620:errorcluster, "handle out"=w619:u32)  [unwired: 3 in, 2 out]
                    n210 = call "Check Rotate Done.vi"("error in (no error)"=w620, "start"=w612, "phandle in"=w619) -> ("error out"=w606:errorcluster)  [unwired: 8 in]
                  }
                  frame "X" {
                    w639 = u16 20039 ("start")
                    n211 = case shown="0" w629 {
                      tunnel: w632 -> [w652 w655]
                      tunnel: [w651 w654] -> w631
                      tunnel: w630 -> [w648 w653]
                      frame Default {
                        n212 = Unbundle By Name(w652) -> ("X Axis.Angle"=w650:dbl)
                        n213 = Add(x=w648, y=w650) -> (x+y=w649:dbl)
                        n214 = Bundle By Name(cluster=w652, "X Axis.Angle"=w649) -> (w651:T3)
                      }
                      frame 0 {
                        n215 = Bundle By Name(cluster=w655, "X Axis.Angle"=w653) -> (w654:T3)
                      }
                    }
                    n216 = call "Z Aux Modbus Set0x.vi"("pdata"=w643, "error in (no error)"=w638, "inum"=u16 8, "start"=u16 20032, "handle"=w644) -> ("error out"=w636:errorcluster, "handle out"=w637:u32)  [unwired: 3 in, 2 out]
                    n217 = call "Delay Time.vi"("error in (no error)"=w636, "Delay(ms)"=u32 30) -> ("error out"=w634:errorcluster)  [unwired: 9 in]
                    n218 = call "Z Aux Modbus Set0x.vi"("pdata"=w645, "error in (no error)"=w634, "inum"=u16 1, "start"=w639, "handle"=w637) -> ("error out"=w647:errorcluster, "handle out"=w646:u32)  [unwired: 3 in, 2 out]
                    n219 = call "Check Rotate Done.vi"("error in (no error)"=w647, "start"=w639, "phandle in"=w646) -> ("error out"=w633:errorcluster)  [unwired: 8 in]
                  }
                  frame "X+Y" {
                    n220 = Unbundle By Name(w660) -> ("X Axis.Angle"=w662:dbl, "Y Axis.Angle"=w661:dbl)
                    n221 = for {
                      tunnel: w670 -> [w686]
                      shift-right: [w685] -> w665
                      shift-left: w671 -> [w687]
                      tunnel: i32[] [20032, 20040] -> [w683] mode=indexing
                      tunnel: w667 -> [w682]
                      tunnel: [w681] -> w666
                      n222 = call "Z Aux Modbus Set0x.vi"("pdata"=w686, "error in (no error)"=w682, "inum"=u16 8, "start"=w683, "handle"=w687) -> ("error out"=w681:errorcluster, "handle out"=w685:u32)  [unwired: 3 in, 2 out]
                    }
                    n223 = call "Delay Time.vi"("error in (no error)"=w666) -> ("error out"=w664:errorcluster)  [unwired: 10 in]
                    n224 = Add(x=w656, y=w662) -> (x+y=w658:dbl)
                    n225 = Add(x=w661, y=w656) -> (x+y=w657:dbl)
                    n226 = for {
                      tunnel: w672 -> [w678]
                      tunnel: w665 -> [w677]
                      tunnel: i32[] [20039, 20047] -> [w675] mode=indexing
                      tunnel: w664 -> [w674]
                      tunnel: [w673] -> w663
                      n227 = call "Z Aux Modbus Set0x.vi"("pdata"=w678, "error in (no error)"=w674, "inum"=u16 1, "start"=w675, "handle"=w677) -> ("error out"=w680:errorcluster, "handle out"=w679:u32)  [unwired: 3 in, 2 out]
                      n228 = call "Check Rotate Done.vi"("error in (no error)"=w680, "start"=w675, "phandle in"=w679) -> ("error out"=w673:errorcluster)  [unwired: 8 in]
                    }
                    n229 = Bundle By Name(cluster=w660, "X Axis.Angle"=w658, "Y Axis.Angle"=w657) -> (w659:T3)
                  }
                }
              }
            }
            n230 = flat-sequence {
              tunnel: w560 -> [w570]
              tunnel: [w570] -> w559
              frame #0 {
                n231 = Wait (ms)(milliseconds to wait=u32 100) -> ()  [unwired: 1 out]
              }
            }
          }
        }
      }
    }
  }
  "error out" <- w21
  "Data OUT" <- w20
